vi "Pack SetOp And Run.vi"(11 "MissionOp Index":i32) -> (3 "Mission Set Op Index and Run Msg out":refnum<class "Mission Set Op Index and Run Msg.lvclass">)   [LabVIEW 2015, in "RDS Mission Controller Actor.lvlib"]
uses:
  RDS Mission Controller Actor.lvlib
  Libraries/RDS Child Messages/Mission Messages/Mission Set Op Index and Run Msg.lvclass
  Libraries/RDS Framework/RDS Message ID.ctl
  Libraries/RDS Framework/RDS Message Class/RDS Message.lvclass/RDS Message.ctl
  Libraries/RDS Child Messages/Mission Messages/Mission Set Op Index and Run Msg.lvclass/Mission Set Op Index and Run Msg.ctl
  Libraries/RDS Framework/RDS Message Class/RDS Message.lvclass
  Libraries/RDS Child Messages/RDS Child Messages.lvlib
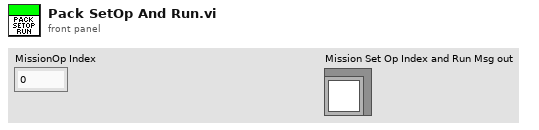
[diagram p1: front panel]
types:
  T1 = typedef "RDS Child Messages.lvlib/RDS Message ID.ctl" = enum16{"RDS Hello World", "String Message", "AIP_Status", "AIP_Command", "GPS_Data", "MCB_Command", "MCB_Status", "Compass_Data", "Depth_Data", "Battery_Data", "Contoller_State", "Set_Mag_Dev", "BTB_Shutdown", "State_Sample_Request", "State_Sample", "PID_Gains_Set", "Helm_Limiter_Set", "Helm_Heading_Command", "Helm_Steering_Command", "Helm_Status", "Controller_Message", "AIP_Set_Min_Depth", "Mission_Controller_State", "Mission_Upload", "Mission_Set_Op_and_Run", "Mission_Settings_Set"}
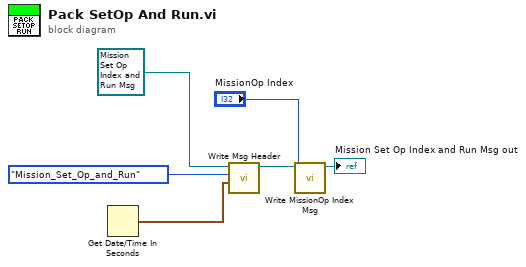
[diagram p0: block diagram]
diagram:
  n1 = Get Date/Time In Seconds() -> (seconds since 1Jan1904=w6:timestamp)
  n2 = call "Write Msg Header.vi"("Time Stamp"=w6, "Msg ID"=RDS_Message_ID."Mission_Set_Op_and_Run", "RDS Message in"=refnum<class "Mission Set Op Index and Run Msg.lvclass"> refnum ("RDS Child Messages.lvlib:Mission Set Op Index and Run Msg.lvclass")) -> ("RDS Message out"=w3:refnum<class "Mission Set Op Index and Run Msg.lvclass">)  [unwired: 7 in, 1 out]
  n3 = call "Write MissionOp Index Msg.vi"("MissionOp Index"="MissionOp Index", "Mission Set Op Index and Run Msg in"=w3) -> ("Mission Set Op Index and Run Msg out"=→"Mission Set Op Index and Run Msg out":refnum<class "Mission Set Op Index and Run Msg.lvclass">)  [unwired: 8 in, 1 out]
